vi "FTW-JSON-Object-GetElement-Bool.vi"(0 "JSON Object":refnum<class "FTW-JSON.lvclass">, 5 "Key":string, 11 "error in":errorcluster) -> (4 "JSON Object out":refnum<class "FTW-JSON.lvclass">, 6 "Value":bool, 8 "Found?":bool, 15 "error out":errorcluster)   [LabVIEW 2013, in "FTW-JSON.lvclass"]
uses:
  FTW-JSON.lvclass
  FTW-JSON.lvclass/FTW-JSON.ctl
  FTW-JSON-Type.ctl
panel:
  # "Inputs"
  # "Outputs"
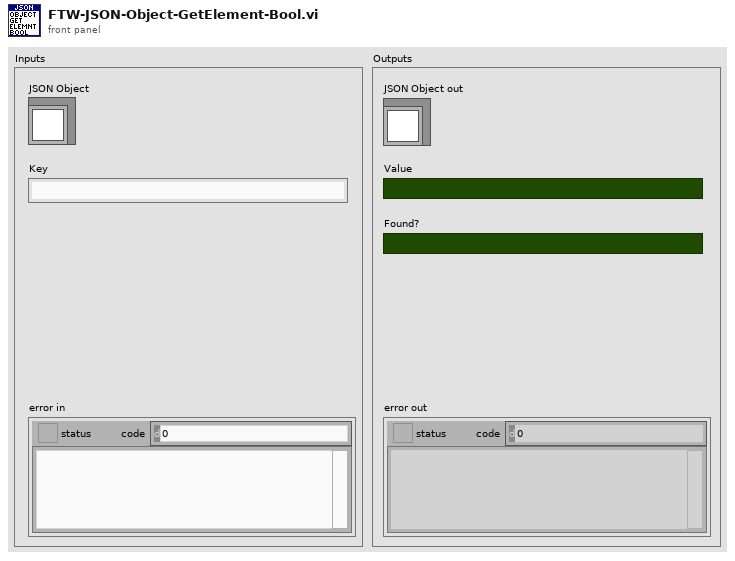
[diagram p1: front panel]
types:
  T1 = typedef "FTW-JSON-Type.ctl" = enum16{"Object", "Array", "String", "Integer", "Floating Point", "true", "false", "null", "undefined"}
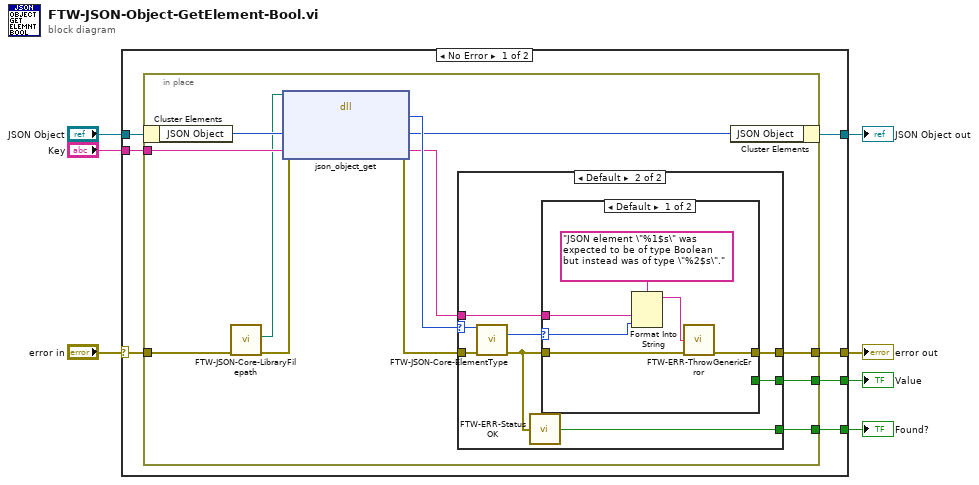
[diagram p0: block diagram]
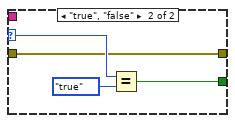
[diagram p3: hidden frame]
diagram:
  n1 = case shown="No Error" "error in" {
    selector: "error in" -> [w14 w47]
    tunnel: [w10 w47] -> w7
    tunnel: [w12 w46] -> w5
    tunnel: "JSON Object" -> [w13 w46]
    tunnel: "Key" -> [w11 _]
    tunnel: [w9 _] -> w2
    tunnel: [w8 _] -> w1
    frame No Error {
      n2 = in-place {
        in-place-border: w14 -> [w26]
        in-place-border: w11 -> [w24]
        in-place-border: [w20] -> w10
        in-place-border: [w19] -> w9
        in-place-border: [w16] -> w8
        n3 = in-place-cluster #1(w13) -> ("JSON Object"=w25:i64)
        n4 = call "FTW-JSON-Core-LibraryFilepath.vi"("error in"=w26) -> ("error out"=w23:errorcluster, "JSON Library Filepath"=w22:path)  [unwired: 9 in]
        n5 = dll-call lib="?" fn="json_object_get"(path in=w22, error in=w23, "JSON Object Pointer"=w25, "Element Key"=w24) -> (error out=w21:errorcluster, "JSON Element Pointer"=w18:i64, "JSON Object Pointer"=w17:i64, "Element Key"=w15:string)  [unwired: 1 in, 1 out]
        n6 = case shown="Default" w18 {
          selector: w18 -> [_ w35]
          tunnel: w21 -> [w27 w31]
          tunnel: [w27 w32] -> w20
          tunnel: [_ w34] -> w19
          tunnel: [_ w29] -> w16
          tunnel: w15 -> [_ w30]
          frame 0 {
          }
          frame Default {
            n7 = call "FTW-JSON-Core-ElementType.vi"("JSON Element"=w35, "error in"=w31) -> ("JSON Type"=w33:T1, "error out"=w28:errorcluster)  [unwired: 11 in, 1 out]
            n8 = call "FTW-ERR-StatusOK.vi"("error to check"=w28) -> ("Status OK?"=w29:bool)
            n9 = case shown="Default" w33 {
              selector: w33 -> [w37 w43]
              tunnel: [_ w44] -> w34
              tunnel: w28 -> [w41 w42]
              tunnel: [w36 w42] -> w32
              tunnel: w30 -> [w38 _]
              frame Default {
                n10 = Format Into String(format string="JSON element \"%1$s\" was expected to be of type Boolean but instead was of type \"%2$s\"." ("Error Message"), w38, w37) -> (resulting string=w39:string)  [unwired: 2 in, 1 out]
                n11 = call "FTW-ERR-ThrowGenericError.vi"("Error Message"=w39, "error in"=w41) -> ("error out"=w36:errorcluster)  [unwired: 13 in]
              }
              frame "true", "false" {
                n12 = Equal?(x=w43, y=FTW-JSON-Type."true" ("x")) -> (x = y?=w44:bool)
              }
            }
          }
        }
        n13 = in-place-cluster #1("JSON Object"=w17) -> (w12:refnum<class "FTW-JSON.lvclass">)
      }
    }
    frame Error {
    }
  }
  "error out" <- w7
  "JSON Object out" <- w5
  "Value" <- w2
  "Found?" <- w1
